vi "vision_webcam_V3_chopped.vi"(11 "dup Message Queue 2":refnum<queue>) -> ()   [LabVIEW 2017]
uses:
  <vilib>/vision/driver/NI_Vision_Acquisition_Software.lvlib
  Globals/Global - All RT Loop Stop.vi
  <vilib>/userdefined/High Color/IMAQdx.ctl
  Globals/Global - Configuration Options.vi
  <vilib>/vision/Image Controls.llb/IMAQ Image.ctl
  Control 2.ctl
  camera_array_1.ctl
  UI Error Handlers/support/Message Queue/Message Cluster.ctl
  UI Error Handlers/support/Message Queue/Message Queue.lvlib
panel:
  out "size(s)":i32
  out "Webcam":T1(plugin-control)
  out "x-y":u32
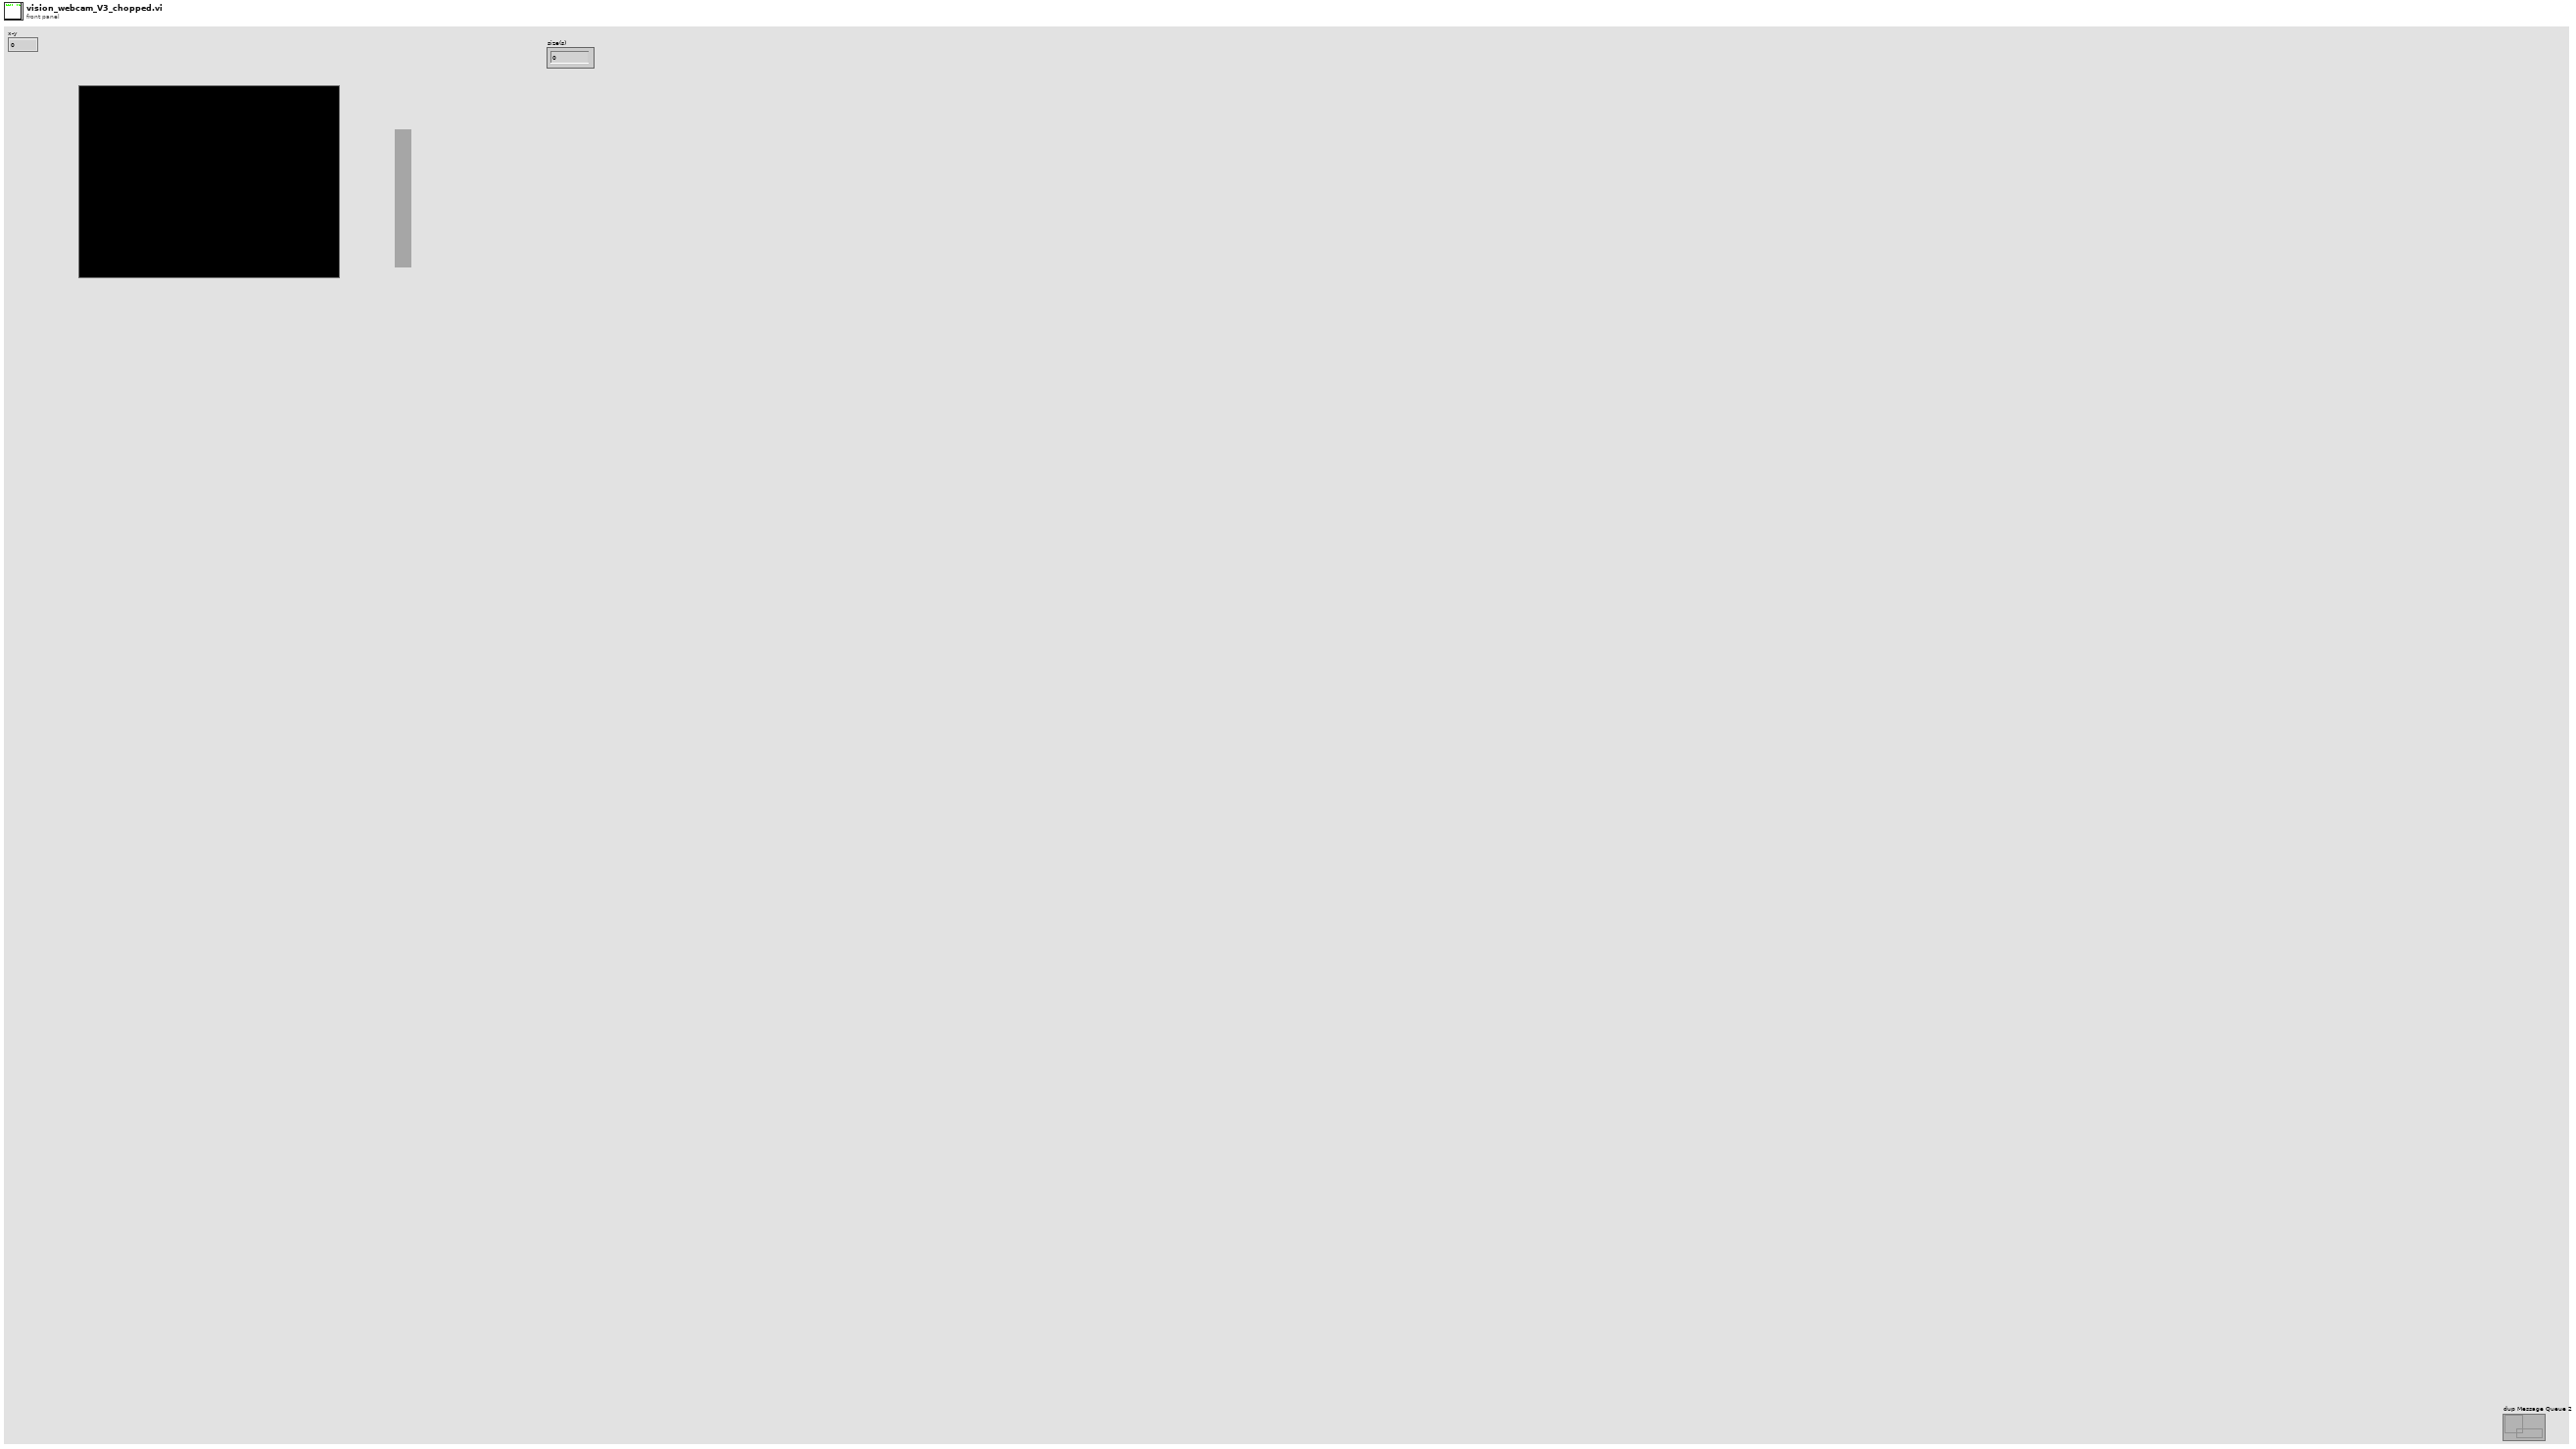
[diagram p1: front panel]
types:
  T1 = typedef "IMAQ Image.ctl" = refnum<image>
  T2 = typedef "Control 2.ctl" = T1[]
  T3 = typedef "IMAQdx.ctl" = refnum<k21>
  T4 = typedef "Image Type" = u32
  T5 = cluster{"Tool data":cluster{"Number of teeth":sgl}, "Cutting data":cluster{"rpm":sgl}, "Limits":cluster{"Magnitude threshold":sgl, "Tolerance":sgl}, "G1 status":cluster{"G1 trigger":bool}}
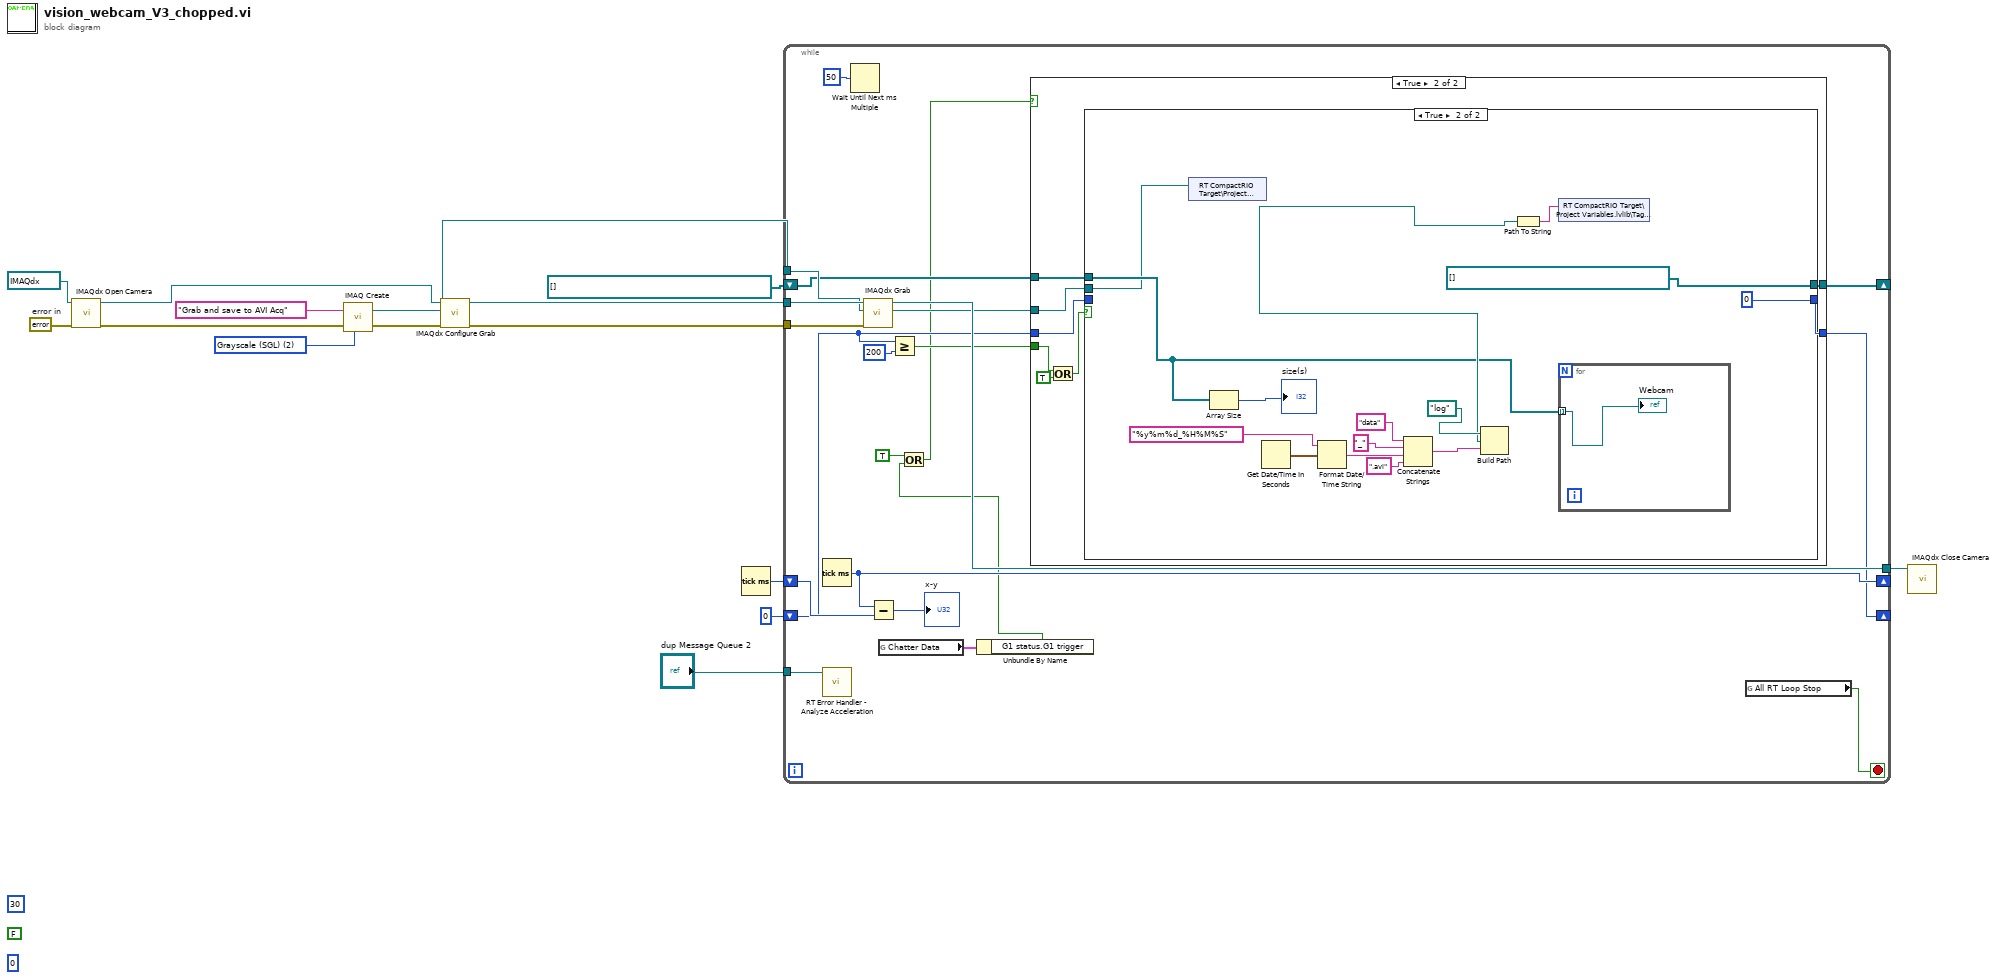
[diagram p0: block diagram]
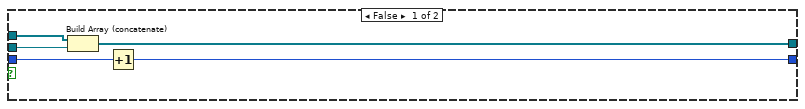
[diagram p3: hidden frame]
diagram:
  w10 = T4 2 items=["Grayscale (U8)", "Grayscale (I16)", "Grayscale (SGL)", "Complex (CSG)", "RGB (U32)", "HSL (U32)", "RGB (U64)", "Grayscale (U16)"] ("Image Type")
  (unwired) u32 30 ("Frames Per Second")
  w11 = errorcluster {"status"=FALSE, "code"=0, "source"=""}  # error in
  (unwired) i16 0 ("A(I16) 11")
  (unwired) FALSE
  n1 = call <vilib>:"IMAQdx Open Camera.vi"("error in"=w11, "Session In"=T3 "cam0") -> ("error out"=w9:errorcluster, "Session Out"=w13:T3)  [unwired: 8 in]
  n2 = call "IMAQ Create"("Image Name"="Grab and save to AVI Acq", "Image Type"=w10, "error in (no error)"=w9) -> ("New Image"=w6:T1, "error out"=w5:errorcluster)  [unwired: 2 in]
  n3 = call <vilib>:"IMAQdx Configure Grab.vi"("error in"=w5, "Session In"=w13) -> ("error out"=w4:errorcluster, "Session Out"=w7:T3)  [unwired: 8 in]
  n4 = Tick Count (ms)() -> (millisecond timer value=w14:u32)
  n5 = while {
    tunnel: "dup Message Queue 2" -> [w36]
    shift-right: [w32] -> _
    shift-left: w14 -> [w33]
    tunnel: w7 -> [w31]
    tunnel: w6 -> [w30]
    tunnel: w4 -> [w29]
    tunnel: [w28] -> w3
    shift-right: [w21] -> _
    shift-left: T2 [] -> [w25]
    shift-right: [w22] -> _
    shift-left: 0 -> [w23]
    stop <- w20 stop-if-true
    n6 = Tick Count (ms)() -> (millisecond timer value=w32:u32)
    n7 = call "RT Error Handler - Analyze Acceleration.vi"("Message Queue"=w36) -> ()  [unwired: 10 in, 1 out]
    n8 = Wait Until Next ms Multiple(millisecond multiple=u32 50) -> ()  [unwired: 1 out]
    n9 = call <vilib>:"IMAQdx Grab.vi"("error in"=w29, "Image In"=w30, "Session In"=w31) -> ("Image Out"=w19:T1, "Session Out"=w28:T3)  [unwired: 5 in, 2 out]
    n10 = Subtract(x=w32, y=w33) -> (x-y=→"x-y":u32)
    n11 = global read "Global - Configuration Options.vi" "Chatter Data"() -> (w35:T5)
    n12 = Greater Or Equal?(x=w23, y=200) -> (x >= y?=w24:bool)
    n13 = Unbundle By Name(w35) -> ("G1 status.G1 trigger"=w18:bool)
    n14 = Or(x=TRUE, y=w18) -> (x .or. y?=w16:bool)
    n15 = case shown="True" w16 {
      tunnel: w19 -> [_ w46]
      tunnel: w25 -> [w37 w45]
      tunnel: w24 -> [_ w41]
      tunnel: w23 -> [w38 w44]
      tunnel: [w38 w43] -> w22
      tunnel: [w37 w42] -> w21
      frame False {
      }
      frame True {
        n16 = Or(x=w41, y=TRUE) -> (x .or. y?=w39:bool)
        n17 = case shown="True" w39 {
          tunnel: w46 -> [w50 w52]
          tunnel: w45 -> [w51 w54]
          tunnel: w44 -> [w49 _]
          tunnel: [w48 0] -> w43
          tunnel: [w47 T2 []] -> w42
          frame False {
            n18 = Build Array (concatenate)(w51, w50) -> (w47:T2)
            n19 = Increment(x=w49) -> (x+1=w48:i32)
          }
          frame True {
            n20 = shared-variable "RT CompactRIO Target\\Project Variables.lvlib\\Images"(w52) -> ()  [unwired: 1 in, 1 out]
            n21 = Array Size(array=w54) -> (size(s)=→"size(s)":i32)
            n22 = Get Date/Time In Seconds() -> (seconds since 1Jan1904=w63:timestamp)
            n23 = Format Date/Time String(time format string (%c)="%y%m%d_%H%M%S", seconds (now)=w63) -> (date/time string=w62:string)  [unwired: 1 out]
            n24 = Concatenate Strings("data" ("string"), "_" ("string"), w62, ".avi" ("string")) -> (w64:string)
            n25 = Build Path(base path=path "log", name or relative path=w64) -> (appended path=w56:path)
            n26 = Path To String(path=w56) -> (string=w66:string)
            n27 = shared-variable "RT CompactRIO Target\\Project Variables.lvlib\\Tag Video"(w66) -> ()  [unwired: 1 in, 1 out]
            n28 = for {
              tunnel: w54 -> [w67] mode=indexing
              "Webcam" <- w67
            }
          }
        }
      }
    }
    n29 = global read "Global - All RT Loop Stop.vi" "All RT Loop Stop"() -> (w20:bool)
  }
  n30 = call <vilib>:"IMAQdx Close Camera.vi"("Session In"=w3) -> ()  [unwired: 10 in, 1 out]
